vi "Get Table Content Pos and Bound.vi"(8 "error in (no error)":errorcluster caption="错误输入（无错误）", 11 "Table Ref In":refnum<vi>) -> (0 "error out":errorcluster caption="错误输出", 1 "内容区域边界":T1, 2 "内容区域位置":T2, 3 "Table Ref Out":refnum<vi>)   [LabVIEW 2013, in "Table Tool.lvlib"]
uses:
  Table Tool.lvlib
  <vilib>/Utility/miscctls.llb/LVPositionTypeDef.ctl
  <vilib>/Utility/miscctls.llb/LVBoundsTypeDef.ctl
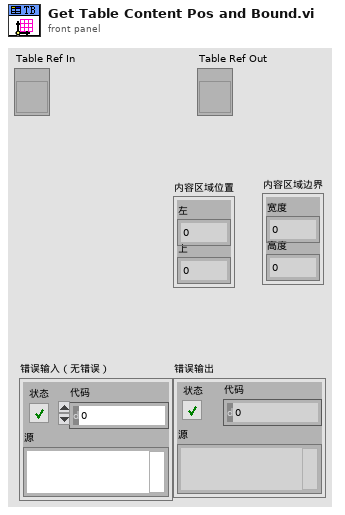
[diagram p1: front panel]
types:
  T1 = typedef "LVBoundsTypeDef.ctl" = cluster{"Width":u32, "Height":u32}
  T2 = typedef "LVPositionTypeDef.ctl" = cluster{"Left":i32, "Top":i32}
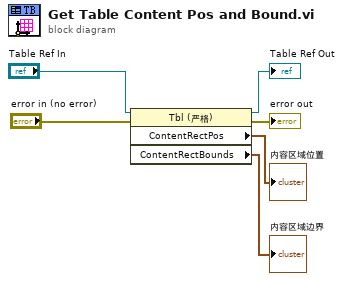
[diagram p0: block diagram]
diagram:
  n1 = property class="Tbl (严格)"(reference="Table Ref In", error in="error in (no error)") -> (reference out=→"Table Ref Out":refnum<vi>, error out=→"error out":errorcluster, "ContentRectPos"=→"内容区域位置":T2, "ContentRectBounds"=→"内容区域边界":T1)
